vi "Report Temperature.vi"(8 "error in (no error)":errorcluster, 10 "Temperature":dbl, 11 "Front Panel Emulator in":refnum<class "Front Panel Emulator.lvclass">) -> (0 "error out":errorcluster, 3 "Front Panel Emulator out":refnum<class "Front Panel Emulator.lvclass">)   [LabVIEW 2020, in "Front Panel Emulator.lvlib" / "Front Panel Emulator.lvclass"]
uses:
  Front Panel Emulator.lvclass
  Front Panel Emulator.lvclass/Front Panel Emulator.ctl
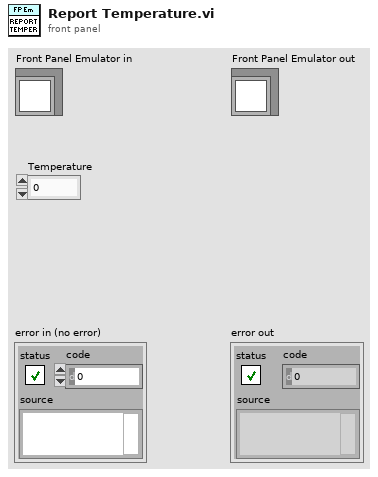
[diagram p1: front panel]
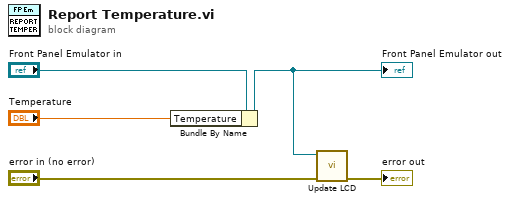
[diagram p0: block diagram]
diagram:
  n1 = Bundle By Name(cluster="Front Panel Emulator in", "Temperature"="Temperature") -> (w2:refnum<class "Front Panel Emulator.lvclass">)
  "Front Panel Emulator out" <- w2
  n2 = call "Update LCD.vi"("error in (no error)"="error in (no error)", "Front Panel Emulator in"=w2) -> ("error out"=→"error out":errorcluster)  [unwired: 9 in]
